vi "Teleop.vi"(10 "Match Info":T1={"Autonomous Elapsed Seconds"=0.0, "TeleOp Elapsed Seconds"=0.0, "Disabled Elapsed Seconds"=0.0, "Visited Autonomous"=FALSE, "Visited TeleOp"=FALSE, "Visited Disabled"=FALSE, "Autonomous Settings"={"Autonomous Style"=enum."Independent", "VI Refnum"=refnum}}, 11 "Call Context":T2) -> ()   [LabVIEW 2015]
doc: "This VI is called for each TeleOp packet received from the DS where the robot is not disabled. It is often used to read from the joysticks and update I/O or to update setpoints for timed control loops. It should complete and return within 20 milliseconds or it may miss DS packets."
uses:
  <vilib>/Rock Robotics/WPI/DriverStation/WPI_DriverStationDerivedRobotMode.ctl
  <vilib>/Rock Robotics/WPI/DriverStation/WPI_DriverStationMatch Info.ctl
  <vilib>/Rock Robotics/WPI/SafetyOutput/WPI_SafetyOutputConfigMenu.ctl
  <vilib>/Rock Robotics/WPI/Utilities/WPI_GetSetVariantRefNum.vi
  <vilib>/Rock Robotics/Network Tables/SD Write Boolean Array.vi
  <vilib>/Rock Robotics/Network Tables/SD Write Numeric Array.vi
  <vilib>/Rock Robotics/Network Tables/NT Read Boolean.vi
  <vilib>/Rock Robotics/WPI/Solenoid/Deprecated/WPI_SolenoidSetBool.vi
  <vilib>/Rock Robotics/WPI/Solenoid/WPI_SolenoidGetEnum.vi
panel:
  out "Claw Closed":bool
  out "X":dbl
  out "Y":dbl
  # "Live Values"
  # "Drive Control"
  # "Lift Control"
  # "Claw Control"
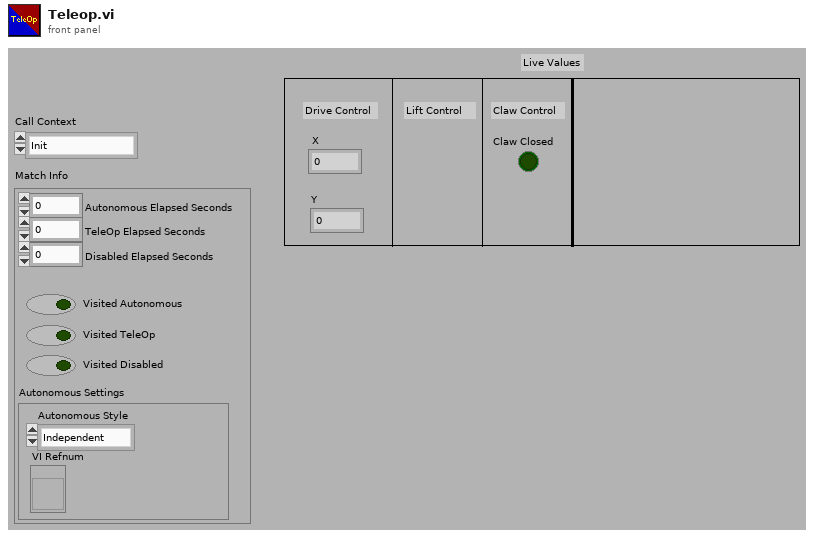
[diagram p1: front panel]
types:
  T1 = typedef "WPI_DriverStationMatch Info.ctl" = cluster{"Autonomous Elapsed Seconds":dbl, "TeleOp Elapsed Seconds":dbl, "Disabled Elapsed Seconds":dbl, "Visited Autonomous":bool, "Visited TeleOp":bool, "Visited Disabled":bool, "Autonomous Settings":cluster{"Autonomous Style":enum16{"Iterative", "Independent"}, "VI Refnum":refnum<vi>}}
  T2 = typedef "WPI_DriverStationDerivedRobotMode.ctl" = enum16{"Init", "Execute", "Stop"}
  T3 = typedef "WPI_SafetyOutputConfigMenu.ctl" = enum16{"Enable", "Disable"}
  T4 = typedef "WPI_CompressorDevRef.ctl" = cluster{"DevStatus":errorcluster, "Pneumatics Control Module":u8}
  T5 = typedef "WPI_SolenoidDevRef.ctl" = cluster{"DevStatus":errorcluster, "Pneumatics Control Module":u8, "Forward Solenoid Channel":T6, "Reverse Solenoid Channel":T6}
  T6 = typedef "WPI_SolenoidChannel.ctl" = enum8{"Solenoid 0", "Solenoid 1", "Solenoid 2", "Solenoid 3", "Solenoid 4", "Solenoid 5", "Solenoid 6", "Solenoid 7", "Invalid"}
  T7 = typedef "WPI_DigitalInputDevRef.ctl" = cluster{"DevStatus":errorcluster, "DIO Channel":T8}
  T8 = typedef "FPGA_DIOChannel.ctl" = enum8{"DIO 0", "DIO 1", "DIO 2", "DIO 3", "DIO 4", "DIO 5", "DIO 6", "DIO 7", "DIO 8", "DIO 9", "DIO MXP 0", "DIO MXP 1", "DIO MXP 2", "DIO MXP 3", "DIO MXP 4", "DIO MXP 5", "DIO MXP 6", "DIO MXP 7", "DIO MXP 8", "DIO MXP 9", "DIO MXP 10", "DIO MXP 11", "DIO MXP 12", "DIO MXP 13", "DIO MXP 14", "DIO MXP 15", "Invalid"}
  T9 = typedef "WPI_JoystickDevRef.ctl" = cluster{"Device":T10}
  T10 = typedef "WPI_JoystickDeviceEnum.ctl" = enum16{"USB 0", "USB 1", "USB 2", "USB 3", "USB 4", "USB 5"}
  T11 = typedef "WPI_RobotDriveDevRef.ctl" = cluster{"DevStatus":errorcluster, "Motors[]":T12[], "Square Inputs":bool, "Max Output":dbl}
  T12 = typedef "WPI_MotorControlDeviceRef.ctl" = cluster{"DeviceStatus":errorcluster, "Type":T13, "PWM":cluster{"PWM Channel":T14, "DeadBand":T15}, "CAN":cluster{"Device Number":u8, "Control Mode":T16, "Semaphore":T17, "Max Vout":dbl, "TalonSRX Control Mode":T18}, "Invert":bool}
  T13 = typedef "WPI_MotorControlType.ctl" = enum16{"PWM", "CAN", "CANTalonSRX"}
  T14 = typedef "FPGA_DIOPWMChannel.ctl" = enum8{"PWM 0", "PWM 1", "PWM 2", "PWM 3", "PWM 4", "PWM 5", "PWM 6", "PWM 7", "PWM 8", "PWM 9", "PWM MXP 0", "PWM MXP 1", "PWM MXP 2", "PWM MXP 3", "PWM MXP 4", "PWM MXP 5", "PWM MXP 6", "PWM MXP 7", "PWM MXP 8", "PWM MXP 9", "Invalid"}
  T15 = typedef "WPI_PWMDeadband.ctl" = cluster{"Name":string, "maxPositivePwm":i32, "minPositivePwm":i32, "centerPwm":i32, "maxNegativePwm":i32, "minNegativePwm":i32, "angularRange":u16}
  T16 = typedef "WPI_CANJaguar_ControlMode.ctl" = enum8{"Percent VBus", "Current", "Speed", "Position", "Voltage"}
  T17 = typedef "Semaphore RefNum" = refnum<k1>
  T18 = typedef "WPI_CANTalonSRX_APIControlMode.ctl" = enum8{"Percent VBus", "Speed", "Position", "Slave", "Unchanged / Invalid", "Voltage Compensation", "Current", "Motion Profile"}
  T19 = cluster{"Axes[0]":dbl, "Axes[1]":dbl, "Axes[2]":dbl, "Axes[3]":dbl, "Axes[4]":dbl, "Axes[5]":dbl, "Axes[6]":dbl, "Axes[7]":dbl, "Axes[8]":dbl}
  T20 = cluster{"Buttons[0]":bool, "Buttons[1]":bool, "Buttons[2]":bool, "Buttons[3]":bool, "Buttons[4]":bool, "Buttons[5]":bool, "Buttons[6]":bool, "Buttons[7]":bool, "Buttons[8]":bool}
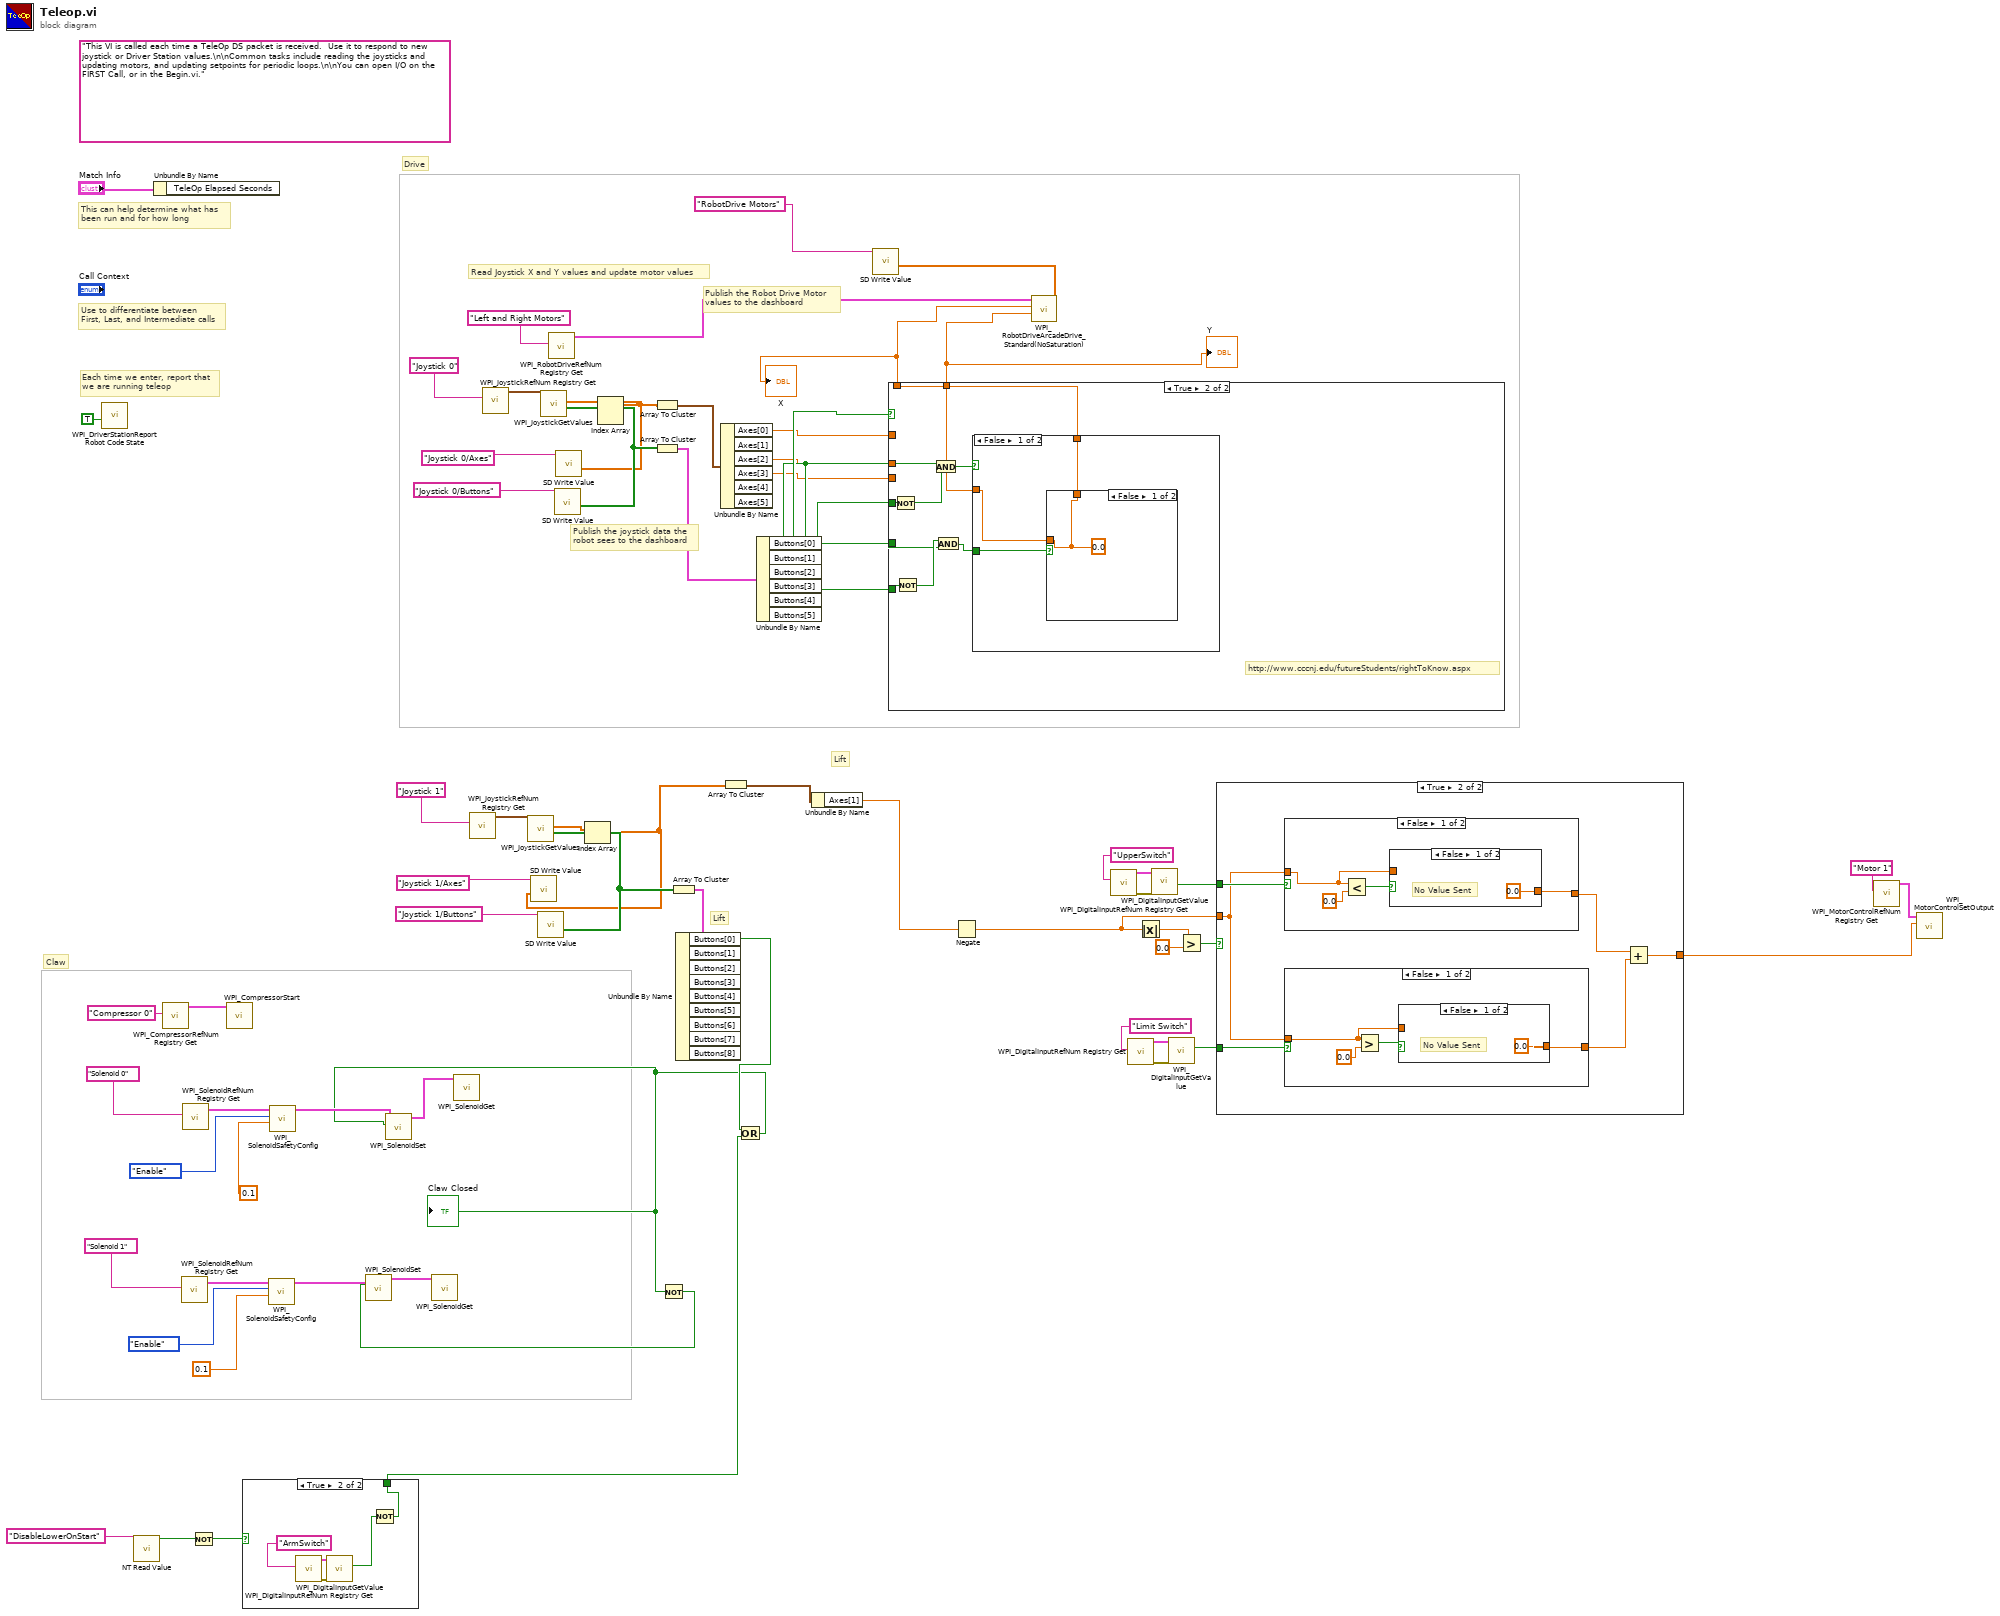
[diagram p0: block diagram]
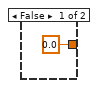
[diagram p2: hidden frame]
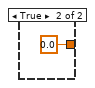
[diagram p4: hidden frame]
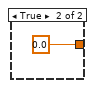
[diagram p6: hidden frame]
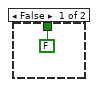
[diagram p7: hidden frame]
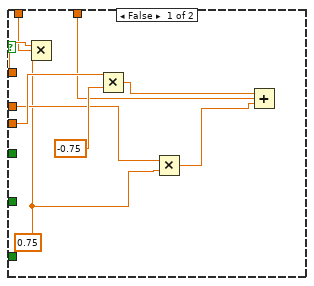
[diagram p8: hidden frame]
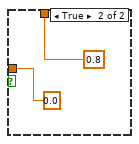
[diagram p9: hidden frame]
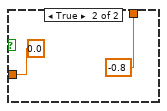
[diagram p10: hidden frame]
diagram:
  (unwired) "This VI is called each time a TeleOp DS packet is received.  Use it to respond to new joystick or Driver Station values.\n\nCommon tasks include reading the joysticks and updating motors, and updating setpoints for periodic loops.\n\nYou can open I/O on the FIRST Call, or in the Begin.vi."
  # "Lift"
  # "Drive"
  # "Claw"
  # "Lift"
  # "Publish the Robot Drive Motor\nvalues to the dashboard"
  # "Publish the joystick data the\nrobot sees to the dashboard"
  # "Each time we enter, report that\nwe are running teleop"
  # "Use to differentiate between\nFirst, Last, and Intermediate calls"
  # "This can help determine what has\nbeen run and for how long"
  # "Read Joystick X and Y values and update motor values"
  n1 = call <vilib>:"WPI_DriverStationReport Robot Code State.vi"("TeleOp"=TRUE ("Autonomous")) -> ()  [unwired: 10 in, 1 out]
  n2 = call-poly <vilib>:"NT Read Value.vi"("Name"="DisableLowerOnStart") -> ("Boolean"=w18:bool)  [unwired: 9 in, 1 out]
  n3 = Unbundle By Name("Match Info") -> ()  [unwired: 1 out]
  n4 = call <vilib>:"WPI_CompressorRefNum Registry Get.vi"("refnum name"="Compressor 0") -> ("CompressorDevRef"=w36:T4)  [unwired: 9 in, 1 out]
  n5 = call <vilib>:"WPI_SolenoidRefNum Registry Get.vi"("refnum name"="Solenoid 1") -> ("SolenoidDevRef"=w33:T5)  [unwired: 9 in, 1 out]
  n6 = call <vilib>:"WPI_SolenoidRefNum Registry Get.vi"("refnum name"="Solenoid 0") -> ("SolenoidDevRef"=w40:T5)  [unwired: 9 in, 1 out]
  n7 = Not(x=w18) -> (.not. x?=w17:bool)
  n8 = call <vilib>:"WPI_CompressorStart.vi"("CompressorDevRef"=w36) -> ()  [unwired: 9 in, 2 out]
  n9 = case shown="True" w17 {
    tunnel: [FALSE ("Value") w69] -> w3
    frame False {
    }
    frame True {
      n10 = call <vilib>:"WPI_DigitalInputRefNum Registry Get.vi"("refnum name"="ArmSwitch") -> ("error out"=w72:errorcluster, "DigitalInputDevRef"=w71:T7)  [unwired: 9 in]
      n11 = call <vilib>:"WPI_DigitalInputGetValue.vi"("error in (no error)"=w72, "DigitalInputDevRef"=w71) -> ("Value"=w70:bool)  [unwired: 7 in, 2 out]
      n12 = Not(x=w70) -> (.not. x?=w69:bool)
    }
  }
  n13 = call <vilib>:"WPI_SolenoidSafetyConfig.vi"("timeout (s)"=0.1, "mode"=WPI_SafetyOutputConfigMenu."Enable", "SolenoidDevRef"=w33) -> ("SolenoidDevRef"=w30:T5)  [unwired: 7 in, 1 out]
  n14 = call <vilib>:"WPI_SolenoidSafetyConfig.vi"("timeout (s)"=0.1, "mode"=WPI_SafetyOutputConfigMenu."Enable", "SolenoidDevRef"=w40) -> ("SolenoidDevRef"=w19:T5)  [unwired: 7 in, 1 out]
  n15 = call <vilib>:"WPI_JoystickRefNum Registry Get.vi"("refnum name"="Joystick 1") -> ("JoystickDevRef"=w46:T9)  [unwired: 1 in, 9 out]
  n16 = call <vilib>:"WPI_JoystickRefNum Registry Get.vi"("refnum name"="Joystick 0") -> ("JoystickDevRef"=w63:T9)  [unwired: 1 in, 9 out]
  n17 = call <vilib>:"WPI_JoystickGetValues.vi"("JoystickDevRef"=w46) -> ("Buttons"=w43:bool[], "Axes"=w28:dbl[])  [unwired: 6 in, 3 out]
  n18 = call-poly <vilib>:"SD Write Value.vi"("Numeric Array"=w28, "Name"="Joystick 1/Axes") -> ()  [unwired: 8 in, 2 out]
  n19 = call-poly <vilib>:"SD Write Value.vi"("Boolean Array"=w43, "Name"="Joystick 1/Buttons") -> ()  [unwired: 8 in, 2 out]
  n20 = call <vilib>:"WPI_JoystickGetValues.vi"("JoystickDevRef"=w63) -> ("Buttons"=w57:bool[], "Axes"=w52:dbl[])  [unwired: 6 in, 3 out]
  n21 = call <vilib>:"WPI_RobotDriveRefNum Registry Get.vi"("refnum name"="Left and Right Motors") -> ("RobotDriveDevRef"=w65:T11)  [unwired: 1 in, 9 out]
  n22 = call-poly <vilib>:"SD Write Value.vi"("Boolean Array"=w57, "Name"="Joystick 0/Buttons") -> ()  [unwired: 8 in, 2 out]
  n23 = call-poly <vilib>:"SD Write Value.vi"("Numeric Array"=w52, "Name"="Joystick 0/Axes") -> ()  [unwired: 8 in, 2 out]
  n24 = Index Array(array=w28) -> ()  [unwired: 1 in, 1 out]
  n25 = Index Array(array=w52) -> ()  [unwired: 2 in, 2 out]
  n26 = Array To Cluster(array=w52) -> (cluster=w51:T19)
  n27 = Array To Cluster(array=w57) -> (cluster=w56:T20)
  n28 = Array To Cluster(array=w43) -> (cluster=w41:T20)
  n29 = Unbundle By Name(w41) -> ("Buttons[0]"=w5:bool)  [unwired: 8 out]
  n30 = Unbundle By Name(w51) -> ("Axes[0]"=w50:dbl, "Axes[2]"=w48:dbl, "Axes[3]"=w49:dbl)  [unwired: 3 out]
  n31 = Array To Cluster(array=w28) -> (cluster=w27:T19)
  n32 = Or(x=w5, y=w3) -> (x .or. y?=w4:bool)
  "Claw Closed" <- w4
  n33 = call-poly <vilib>:"WPI_SolenoidSet.vi"("Value"=w4, "SolenoidDevRef"=w19) -> ("SolenoidDevRef"=w35:T5)  [unwired: 8 in, 1 out]
  n34 = call-poly <vilib>:"WPI_SolenoidGet.vi"("SolenoidDevRef"=w35) -> ()  [unwired: 8 in, 3 out]
  n35 = Not(x=w4) -> (.not. x?=w25:bool)
  n36 = call-poly <vilib>:"WPI_SolenoidSet.vi"("Value"=w25, "SolenoidDevRef"=w30) -> ("SolenoidDevRef"=w29:T5)  [unwired: 8 in, 1 out]
  n37 = call-poly <vilib>:"WPI_SolenoidGet.vi"("SolenoidDevRef"=w29) -> ()  [unwired: 8 in, 3 out]
  n38 = Unbundle By Name(w56) -> ("Buttons[0]"=w55:bool, "Buttons[4]"=w54:bool, "Buttons[5]"=w53:bool)  [unwired: 3 out]
  n39 = Unbundle By Name(w27) -> ("Axes[1]"=w2:dbl)
  n40 = case shown="True" w55 {
    tunnel: [w79 w91] -> w6
    tunnel: [w74 w92] -> w7
    tunnel: w54 -> [_ w87]
    tunnel: w53 -> [_ w83]
    tunnel: w54 -> [_ w86]
    tunnel: w53 -> [_ w85]
    tunnel: w50 -> [w81 _]
    tunnel: w49 -> [w82 _]
    tunnel: w48 -> [w78 _]
    frame False {
      w77 = 0.75 ("y")
      n41 = Multiply(x=w81, y=w77) -> (x*y=w79:dbl)
      n42 = Multiply(x=w82, y=-0.75) -> (x*y=w75:dbl)
      n43 = Multiply(x=w78, y=w77) -> (x*y=w76:dbl)
      n44 = Add(x=w75, y=w76) -> (x+y=w74:dbl)
    }
    frame True {
      # "http://www.cccnj.edu/futureStudents/rightToKnow.aspx"
      n45 = Not(x=w85) -> (.not. x?=w90:bool)
      n46 = Not(x=w87) -> (.not. x?=w84:bool)
      n47 = And(x=w86, y=w90) -> (x .and. y?=w89:bool)
      n48 = And(x=w84, y=w83) -> (x .and. y?=w88:bool)
      n49 = case shown="False" w89 {
        tunnel: [w95 0.0] -> w92
        tunnel: [w94 -0.8] -> w91
        tunnel: w88 -> [w93 _]
        frame False {
          n50 = case shown="False" w93 {
            tunnel: [w96 0.0] -> w95
            tunnel: [w96 0.8] -> w94
            frame False {
              w96 = 0.0
            }
            frame True {
            }
          }
        }
        frame True {
        }
      }
    }
  }
  "Y" <- w7
  "X" <- w6
  n51 = Negate(x=w2) -> (-x=w1:dbl)
  n52 = call <vilib>:"WPI_RobotDriveArcadeDrive_Standard(NoSaturation).vi"("Y axis value"=w7, "X axis value"=w6, "RobotDriveDevRef"=w65) -> ("Motor Values"=w60:dbl[])  [unwired: 1 in, 7 out]
  n53 = call-poly <vilib>:"SD Write Value.vi"("Numeric Array"=w60, "Name"="RobotDrive Motors") -> ()  [unwired: 8 in, 2 out]
  n54 = call <vilib>:"WPI_DigitalInputRefNum Registry Get.vi"("refnum name"="UpperSwitch") -> ("error out"=w13:errorcluster, "DigitalInputDevRef"=w14:T7)  [unwired: 9 in]
  n55 = call <vilib>:"WPI_DigitalInputRefNum Registry Get.vi"("refnum name"="Limit Switch") -> ("error out"=w21:errorcluster, "DigitalInputDevRef"=w22:T7)  [unwired: 9 in]
  n56 = Absolute Value(x=w1) -> (abs(x)=w11:dbl)
  n57 = call <vilib>:"WPI_DigitalInputGetValue.vi"("error in (no error)"=w13, "DigitalInputDevRef"=w14) -> ("Value"=w12:bool)  [unwired: 7 in, 2 out]
  n58 = call <vilib>:"WPI_DigitalInputGetValue.vi"("error in (no error)"=w21, "DigitalInputDevRef"=w22) -> ("Value"=w16:bool)  [unwired: 7 in, 2 out]
  n59 = Greater?(x=w11, y=0.0) -> (0:w9:bool)
  n60 = case shown="True" w9 {
    tunnel: w16 -> [_ w107]
    tunnel: w12 -> [_ w106]
    tunnel: [0.0 w105] -> w8
    tunnel: w1 -> [_ w102]
    frame False {
    }
    frame True {
      n61 = case shown="False" w106 {
        tunnel: [w111 0.0 ("x")] -> w104
        tunnel: w102 -> [w108 _]
        frame False {
          n62 = Less?(x=w108, y=0.0) -> (x < y?=w110:bool)
          n63 = case shown="False" w110 {
            tunnel: [0.0 ("y") w113] -> w111
            tunnel: w108 -> [_ w113]
            frame False {
              # "No Value Sent"
            }
            frame True {
            }
          }
        }
        frame True {
        }
      }
      n64 = case shown="False" w107 {
        tunnel: [w118 0.0 ("y")] -> w103
        tunnel: w102 -> [w115 _]
        frame False {
          n65 = Greater?(x=w115, y=0.0) -> (0:w117:bool)
          n66 = case shown="False" w117 {
            tunnel: [0.0 ("y") w120] -> w118
            tunnel: w115 -> [_ w120]
            frame False {
              # "No Value Sent"
            }
            frame True {
            }
          }
        }
        frame True {
        }
      }
      n67 = Add(x=w104, y=w103) -> (x+y=w105:dbl)
    }
  }
  n68 = call <vilib>:"WPI_MotorControlRefNum Registry Get.vi"("refnum name"="Motor 1") -> ("MotorControlDevRef"=w24:T12)  [unwired: 9 in, 1 out]
  n69 = call <vilib>:"WPI_MotorControlSetOutput.vi"("Output"=w8, "MotorControlDevRef"=w24) -> ()  [unwired: 7 in, 3 out]
